vi "locate CDs.vi"(8 "error in (no error)":errorcluster, 10 "include files in":variant, 11 "cds":variant=variant("382db339-b6fb-45a6-86c0-031bb1110bb1"=variant(string "382db339-b6fb-45a6-86c0-031bb1110bb1"))) -> (0 "error out":errorcluster, 2 "include files out":variant)   [LabVIEW 2014]
uses:
  <vilib>/Utility/sysdir.llb/System Directory Type.ctl
  <vilib>/xml/Load XML File.vi
  <vilib>/xml/Close Reference(Node).vi
  <vilib>/xml/NI_XML.lvlib
  <resource>/objmgr/DOMUserDefRef.rc
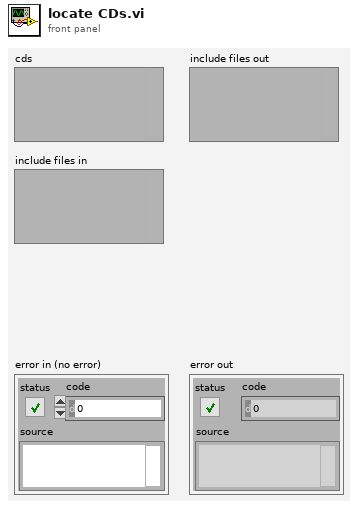
[diagram p1: front panel]
types:
  T1 = typedef "System Directory Type.ctl" = i32
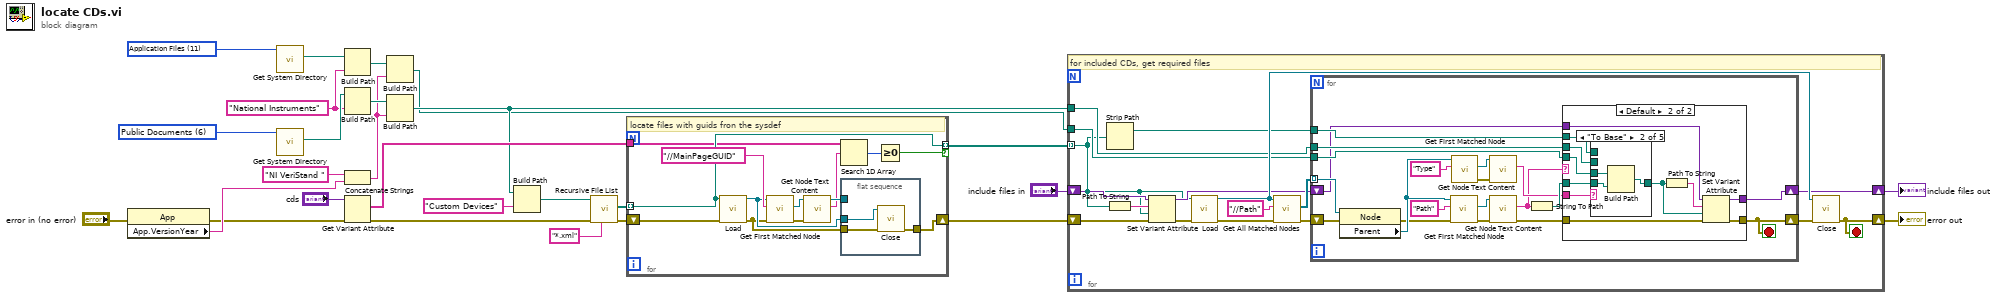
[diagram p0: block diagram]
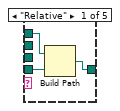
[diagram p3: hidden frame]
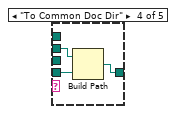
[diagram p5: hidden frame]
diagram:
  w11 = T1 11 items=["User Home"=0, "User Desktop"=1, "User Documents"=2, "User Application Data"=3, "User Preferences"=4, "User Temporary"=5, "Public Documents"=6, "Public Application Data"=7, "Public Preferences"=8, "Public Cache"=13, "System Core Libraries"=9, "System Installed Libraries"=10, "Application Files"=11, "Boot Volume Root"=12] ("system directory type")
  w6 = "National Instruments"
  w27 = T1 6 items=["User Home"=0, "User Desktop"=1, "User Documents"=2, "User Application Data"=3, "User Preferences"=4, "User Temporary"=5, "Public Documents"=6, "Public Application Data"=7, "Public Preferences"=8, "Public Cache"=13, "System Core Libraries"=9, "System Installed Libraries"=10, "Application Files"=11, "Boot Volume Root"=12] ("system directory type")
  n1 = property class="App"(error in="error in (no error)") -> (error out=w14:errorcluster, "App.VersionYear"=w24:string)  [unwired: 1 in, 1 out]
  n2 = call <vilib>:"Get System Directory.vi"("system directory type"=w11) -> ("system directory"=w10:path)  [unwired: 10 in]
  n3 = call <vilib>:"Get System Directory.vi"("system directory type"=w27) -> ("system directory"=w26:path)  [unwired: 10 in]
  n4 = Build Path(base path=w10, name or relative path=w6) -> (appended path=w9:path)
  n5 = Build Path(base path=w26, name or relative path=w6) -> (appended path=w25:path)
  n6 = Concatenate Strings("NI VeriStand ", w24) -> (w8:string)
  n7 = Get Variant Attribute(Variant="cds", error in=w14) -> (names=w17:string[], error out=w16:errorcluster)  [unwired: 2 in, 2 out]
  n8 = Build Path(base path=w9, name or relative path=w8) -> (appended path=w4:path)
  n9 = Build Path(base path=w25, name or relative path=w8) -> (appended path=w5:path)
  n10 = Build Path(base path=w5, name or relative path="Custom Devices") -> (appended path=w7:path)
  n11 = call <vilib>:"Recursive File List.vi"("pattern"="*.xml", "error in (no error)"=w16, "Folder Path"=w7) -> ("error out"=w20:errorcluster, "All Files in Dir"=w19:path[])  [unwired: 4 in, 3 out]
  n12 = for {
    shift-right: [w36] -> w12
    shift-left: w20 -> [w40]
    tunnel: w19 -> [w35] mode=indexing
    tunnel: [w35] -> w13 mode=indexing if=w29
    tunnel: w17 -> [w31]
    # "locate files with guids fron the sysdef"
    n13 = call-poly <vilib>:"Load.vi"("path to XML document"=w35, "error in (no error)"=w40) -> ("DOM document out"=w37:refnum<k20>, "error out"=w33:errorcluster)  [unwired: 11 in, 1 out]
    n14 = call <vilib>:"Get First Matched Node.vi"("error in (no error)"=w33, "XPath expression"="//MainPageGUID", "node in"=w37) -> ("error out"=w38:errorcluster, "node result"=w34:refnum<k20>)  [unwired: 6 in, 1 out]
    n15 = call <vilib>:"Get Node Text Content.vi"("error in (no error)"=w38, "node in"=w34) -> ("node text"=w30:string, "node out"=w32:refnum<k20>)  [unwired: 7 in, 1 out]
    n16 = Search 1D Array(1D array=w31, element=w30) -> (index of element=w28:i32)  [unwired: 1 in]
    n17 = flat-sequence {
      tunnel: w37 -> [w43]
      tunnel: [w42] -> w36
      tunnel: w33 -> [w41]
      tunnel: w32 -> [_]
      frame #0 {
        n18 = call-poly <vilib>:"Close.vi"("error in (no error)"=w41, "node"=w43) -> ("error out"=w42:errorcluster)  [unwired: 7 in]
      }
    }
    n19 = Greater Or Equal To 0?(x=w28) -> (x >= 0?=w29:bool)
  }
  n20 = for {
    tunnel: w13 -> [w44] mode=indexing
    shift-right: [w49] -> w1
    shift-left: w12 -> [w60]
    tunnel: w5 -> [w53]
    tunnel: w4 -> [w52]
    shift-right: [w51] -> w2
    shift-left: "include files in" -> [w47]
    stop <- w49 stop-if-true
    # "for included CDs, get required files"
    n21 = Path To String(path=w44) -> (string=w45:string)
    n22 = Strip Path(path=w44) -> (stripped path=w54:path)  [unwired: 1 out]
    n23 = Set Variant Attribute(Variant=w47, name=w45, value=w44, error in=w60) -> (Variant out=w46:variant, error out=w48:errorcluster)  [unwired: 1 out]
    n24 = call-poly <vilib>:"Load.vi"("path to XML document"=w44, "error in (no error)"=w48) -> ("DOM document out"=w59:refnum<k20>, "error out"=w58:errorcluster)  [unwired: 11 in, 1 out]
    n25 = call <vilib>:"Get All Matched Nodes.vi"("error in (no error)"=w58, "XPath expression"="//Path", "node in"=w59) -> ("error out"=w56:errorcluster, "node result array"=w55:refnum<k20>[])  [unwired: 6 in, 1 out]
    n26 = for {
      tunnel: w55 -> [w79] mode=indexing
      tunnel: w54 -> [w77]
      tunnel: w53 -> [w76]
      tunnel: w52 -> [w75]
      shift-right: [w73] -> w51
      shift-left: w46 -> [w72]
      shift-right: [w61] -> w50
      shift-left: w56 -> [w80]
      stop <- w61 stop-if-true
      n27 = property class="Node"(reference=w79, error in=w80) -> (error out=w74:errorcluster, "Parent"=w78:refnum<k20>)  [unwired: 1 out]
      n28 = call <vilib>:"Get First Matched Node.vi"("error in (no error)"=w74, "XPath expression"="Path", "node in"=w78) -> ("error out"=w64:errorcluster, "node result"=w63:refnum<k20>)  [unwired: 6 in, 1 out]
      n29 = call <vilib>:"Get First Matched Node.vi"("XPath expression"="Type", "node in"=w78) -> ("error out"=w67:errorcluster, "node result"=w68:refnum<k20>)  [unwired: 7 in, 1 out]
      n30 = call <vilib>:"Get Node Text Content.vi"("error in (no error)"=w67, "node in"=w68) -> ("node text"=w66:string)  [unwired: 7 in, 2 out]
      n31 = call <vilib>:"Get Node Text Content.vi"("error in (no error)"=w64, "node in"=w63) -> ("error out"=w62:errorcluster, "node text"=w65:string)  [unwired: 7 in, 1 out]
      n32 = String To Path(string=w65) -> (path=w69:path)
      n33 = case shown="Default" w65 {
        tunnel: w66 -> [_ w93]
        tunnel: w69 -> [_ w92]
        tunnel: w77 -> [_ w91]
        tunnel: w76 -> [_ w90]
        tunnel: w62 -> [w82 w88]
        tunnel: [w82 w89] -> w61
        tunnel: w72 -> [w81 w85]
        tunnel: [w81 w84] -> w73
        tunnel: w75 -> [_ w83]
        frame "" {
        }
        frame Default {
          n34 = case shown="\"To Base\"" w93 {
            tunnel: [w95 w99 w100 w101 w104] -> w87
            tunnel: w92 -> [w94 w98 w100 w102 w104]
            tunnel: w91 -> [w96 _ _ _ _]
            tunnel: w90 -> [_ _ _ w103 _]
            tunnel: w83 -> [_ w97 _ _ _]
            frame "Relative" {
              n35 = Build Path(base path=w96, name or relative path=w94) -> (appended path=w95:path)
            }
            frame "To Base" {
              n36 = Build Path(base path=w97, name or relative path=w98) -> (appended path=w99:path)
            }
            frame "Absolute" {
            }
            frame "To Common Doc Dir" {
              n37 = Build Path(base path=w103, name or relative path=w102) -> (appended path=w101:path)
            }
            frame "", Default {
            }
          }
          n38 = Path To String(path=w87) -> (string=w86:string)
          n39 = Set Variant Attribute(Variant=w85, name=w86, value=w87, error in=w88) -> (Variant out=w84:variant, error out=w89:errorcluster)  [unwired: 1 out]
        }
      }
    }
    n40 = call-poly <vilib>:"Close.vi"("error in (no error)"=w50, "node"=w59) -> ("error out"=w49:errorcluster)  [unwired: 7 in]
  }
  "include files out" <- w2
  "error out" <- w1
